vi "KEYBOARD.vi"() -> (4 "String":string)   [LabVIEW 2014, in "Master.lvclass"]
uses:
  Master/Master.lvclass
panel:
  in  "Tab Control":enum32{"Page 1", "Page 2"}(tab)
  in  "Enter":bool
  in  "Clear":bool
  in  "z":bool
  in  "y":bool
  in  "x":bool
  in  "w":bool
  in  "v":bool
  in  "u":bool
  in  "t":bool
  in  "s":bool
  in  "r":bool
  in  "p":bool
  in  "o":bool
  in  "n":bool
  in  "m":bool
  in  "l":bool
  in  "k":bool
  in  "j":bool
  in  "i":bool
  in  "h":bool
  in  "g":bool
  in  "f":bool
  in  "e":bool
  in  "d":bool
  in  "c":bool
  in  "b":bool
  in  "a":bool
  in  "1":bool
  in  "2":bool
  in  "3":bool
  in  "4":bool
  in  "5":bool
  in  "6":bool
  in  "7":bool
  in  "8":bool
  in  "9":bool
  in  "0":bool
  in  "DEL":bool
  in  "q":bool
  in  "Space":bool
  in  "String (in)":string
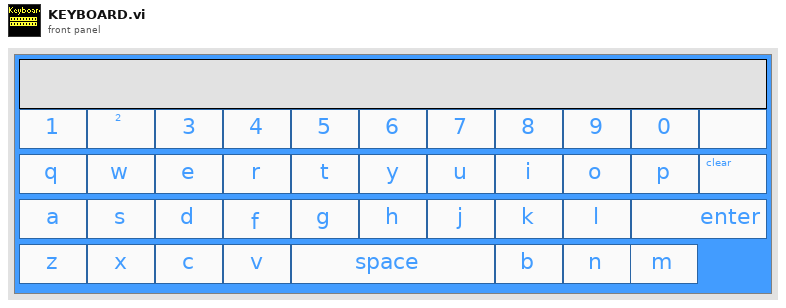
[diagram p1: front panel]
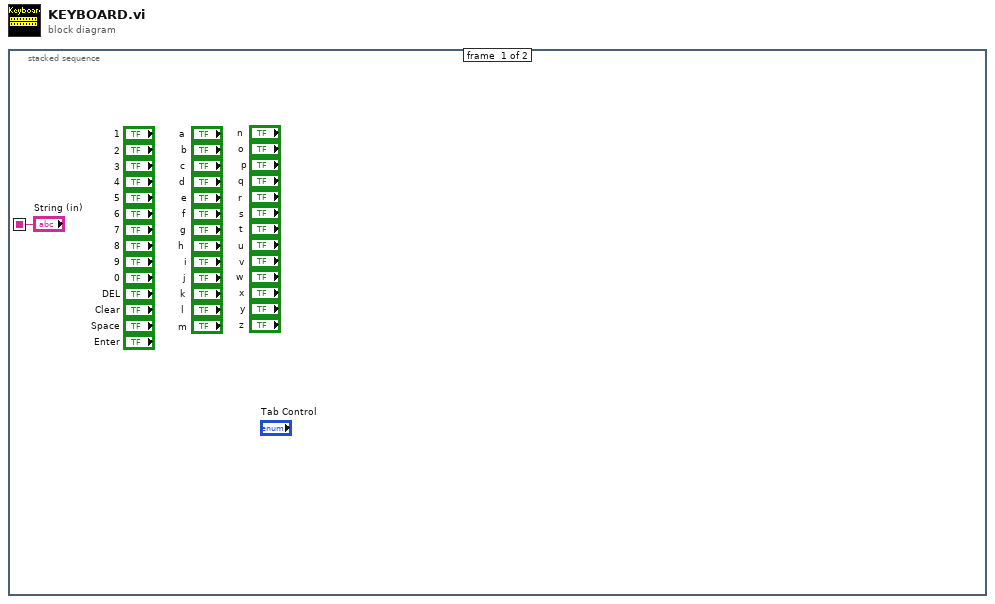
[diagram p0: block diagram]
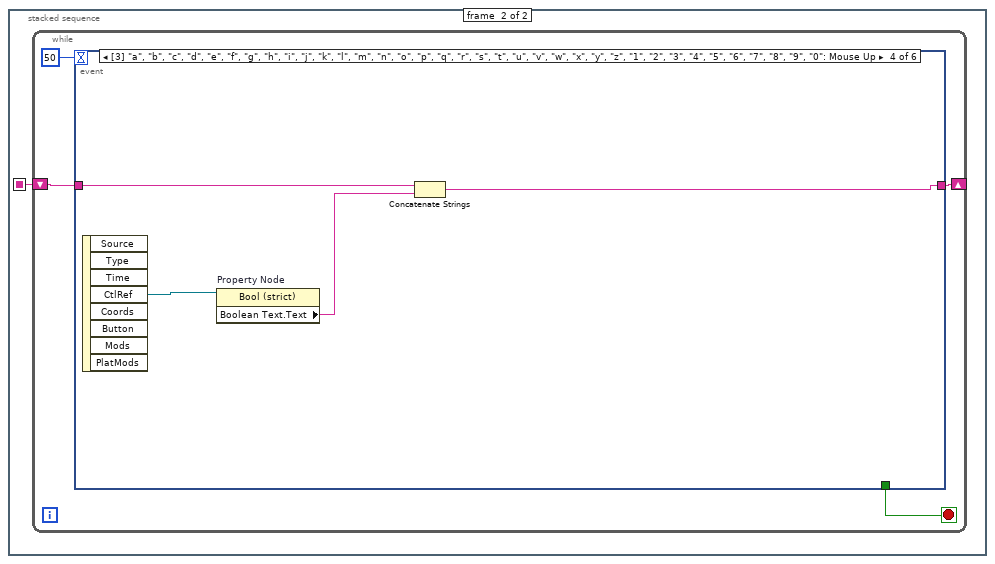
[diagram p2: hidden frame]
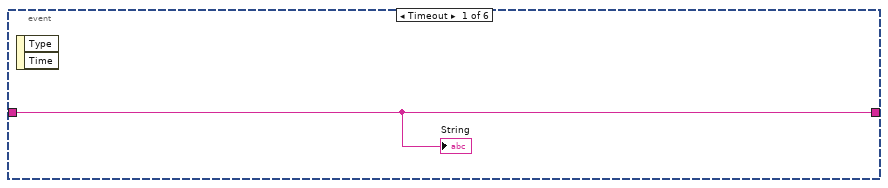
[diagram p3: hidden frame]
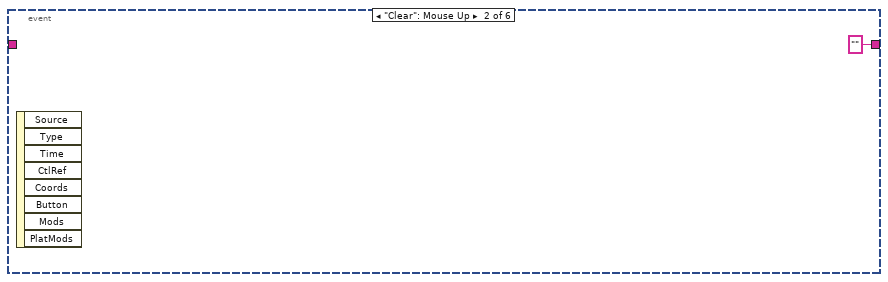
[diagram p4: hidden frame]
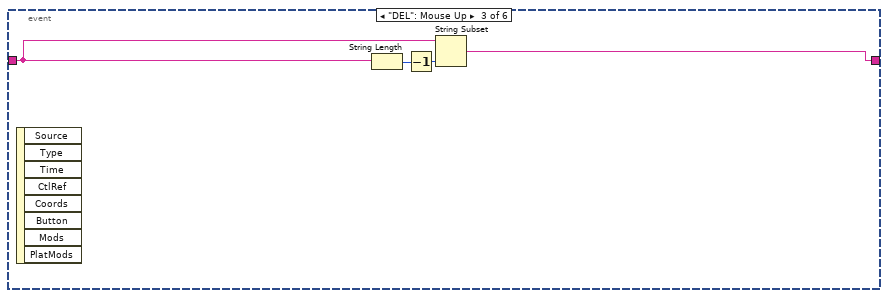
[diagram p5: hidden frame]
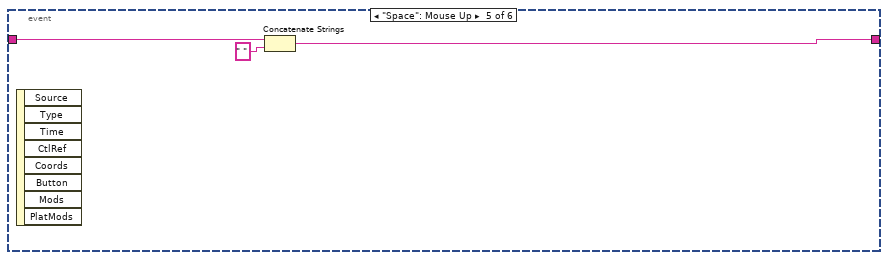
[diagram p6: hidden frame]
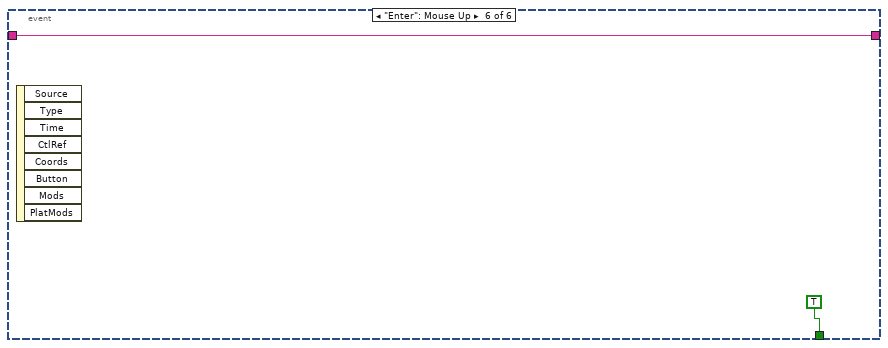
[diagram p7: hidden frame]
diagram:
  n1 = stacked-sequence {
    seq-local: ["String (in)" _] -> [_ w2]
    frame #0 {
    }
    frame #1 {
      n2 = while {
        shift-right: [w5] -> _
        shift-left: w2 -> [w6]
        stop <- w4 stop-if-true
        n3 = event shown="[3] \"a\", \"b\", \"c\", \"d\", \"e\", \"f\", \"g\", \"h\", \"i\", \"j\", \"k\", \"l\", \"m\", \"n\", \"o\", \"p\", \"q\", \"r\", \"s\", \"t\", \"u\", \"v\", \"w\", \"x\", \"y\", \"z\", \"1\", \"2\", \"3\", \"4\", \"5\", \"6\", \"7\", \"8\", \"9\", \"0\": Mouse Up" {
          selector: _ -> [_ _ _ _ _ _]
          dyn-events: _ -> [_ _ _ _ _ _]
          timeout: 50 -> [_ _ _ _ _ _]
          tunnel: w6 -> [w7 _ w12 w16 w19 w20]
          tunnel: [w7 "" w9 w15 w17 w20] -> w5
          tunnel: [_ _ _ _ _ TRUE] -> w4
          event Timeout {
            n4 = event-data() -> ()  [unwired: 1 in, 2 out]
            "String" <- w7
          }
          event "Clear": Mouse Up {
            n5 = event-data() -> ()  [unwired: 1 in, 8 out]
          }
          event "DEL": Mouse Up {
            n6 = event-data() -> ()  [unwired: 1 in, 8 out]
            n7 = String Length(string=w12) -> (length=w11:i32)
            n8 = Decrement(x=w11) -> (x-1=w10:i32)
            n9 = String Subset(string=w12, length (rest)=w10) -> (substring=w9:string)  [unwired: 1 in]
          }
          event "a", "b", "c", "d", "e", "f", "g", "h", "i", "j", "k", "l", "m", "n", "o", "p", "q", "r", "s", "t", "u", "v", "w", "x", "y", "z", "1", "2", "3", "4", "5", "6", "7", "8", "9", "0": Mouse Up {
            n10 = event-data() -> ("CtlRef"=w14:refnum<vi>)  [unwired: 1 in, 7 out]
            n11 = property on="Property Node" class="Bool (strict)"(reference=w14) -> ("Boolean Text.Text"=w13:string)  [unwired: 1 in, 2 out]
            n12 = Concatenate Strings "Concatenate Strings"(w16, w13) -> (w15:string)
          }
          event "Space": Mouse Up {
            n13 = event-data() -> ()  [unwired: 1 in, 8 out]
            n14 = Concatenate Strings(w19, " ") -> (w17:string)
          }
          event "Enter": Mouse Up {
            n15 = event-data() -> ()  [unwired: 1 in, 8 out]
          }
        }
      }
    }
  }
